vi "Initialize.vi"(8 "error in (no error)":errorcluster, 11 "GSserver in":refnum<class "GSserver.lvclass">) -> (0 "error out":errorcluster, 3 "GSserver out":refnum<class "GSserver.lvclass">)   [LabVIEW 2018, in "GSserver.lvclass"]
uses:
  GSserver.lvclass
  C:/Users/devstaff/sparc4/s4gui/Versao ZeroMQ REQ-REP/SPARC4_GUI -v1.0.8 - reconhecimento do ACK do ACS/Server/Server.lvclass
  GSserver.lvclass/GSserver.ctl
  Server/Server.lvclass/Server.ctl
  GSdevice/GSdevice.lvclass
  Server/Server.lvclass
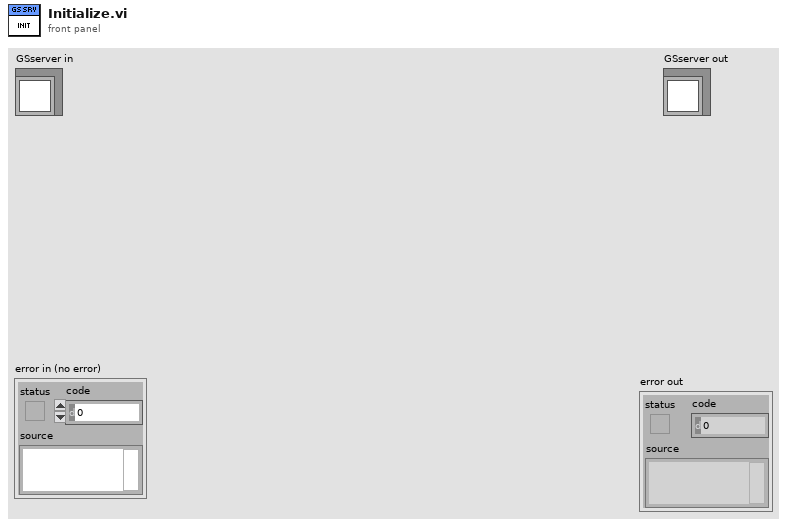
[diagram p1: front panel]
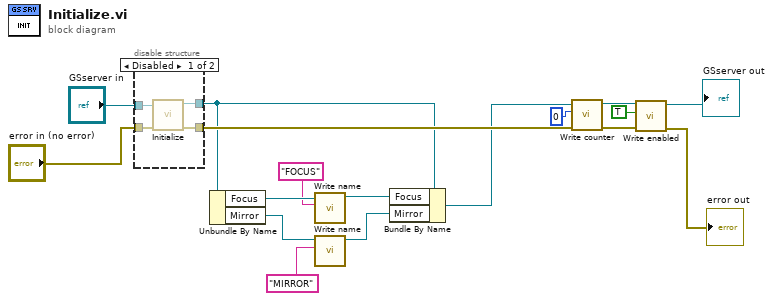
[diagram p0: block diagram]
diagram:
  n1 = disable-structure shown="Disabled" {
    disable-tunnel: [w21 w22] -> w11
    disable-tunnel: [w20 w23] -> w4
    disable-tunnel: "error in (no error)" -> [w19 w22]
    disable-tunnel: "GSserver in" -> [w18 w23]
    frame Disabled {
      n2 = call-parent "Initialize.vi"("error in (no error)"=w19, "Server in"=w18) -> ("error out"=w21:errorcluster, "Server out"=w20:refnum<class "GSserver.lvclass">)  [unwired: 8 in]
    }
    frame Enabled {
    }
  }
  n3 = Unbundle By Name(w4) -> ("Focus"=w8:refnum<class "GSdevice.lvclass">, "Mirror"=w7:refnum<class "GSdevice.lvclass">)
  n4 = call-dynamic "Write name.vi"("name"="FOCUS", "GSdevice in"=w8) -> ("GSdevice out"=w2:refnum<class "GSdevice.lvclass">)  [unwired: 8 in, 1 out]
  n5 = call-dynamic "Write name.vi"("name"="MIRROR", "GSdevice in"=w7) -> ("GSdevice out"=w1:refnum<class "GSdevice.lvclass">)  [unwired: 8 in, 1 out]
  n6 = Bundle By Name(cluster=w4, "Focus"=w2, "Mirror"=w1) -> (w3:refnum<class "GSserver.lvclass">)
  n7 = call "Write counter.vi"("error in (no error)"=w11, "counter"=u32 0, "Server in"=w3) -> ("error out"=w10:errorcluster, "Server out"=w15:refnum<class "GSserver.lvclass">)  [unwired: 7 in]
  n8 = call-dynamic "Write enabled.vi"("error in (no error)"=w10, "enabled"=TRUE, "Server in"=w15) -> ("error out"=→"error out":errorcluster, "Server out"=→"GSserver out":refnum<class "GSserver.lvclass">)  [unwired: 7 in]
